vi "SPINUPGUN.vi"(10 "argv":string[](array[string]), 11 "args":u8) -> ()   [LabVIEW 2011]
uses:
  <vilib>/Rock Robotics/WPI/DriverStation/WPI_DriverStationStatusErrorCache.ctl
  signals/Signal.ctl
  Auto_Conf.vi
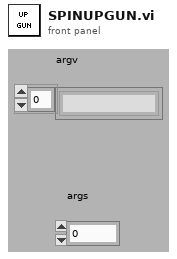
[diagram p1: front panel]
types:
  T1 = typedef "Signal.ctl" = enum16{"SIGFIRE", "SIGSTOPSCRIPT", "SIGSTARTGUN", "SIGSTOPGUN", "SIGDISABLED", "SIGENABLED", "SIGUDPTIMEOUT", "SIGNEWVISION_REMOTE", "SIGNEWVISION_LOCAL", "SIGSHOTFIRED", "SIGDOTRACK", "SIGDONTTRACK"}
  T2 = typedef "WPI_DriverStationStatusErrorCache.ctl" = enum16{"Get", "Set"}
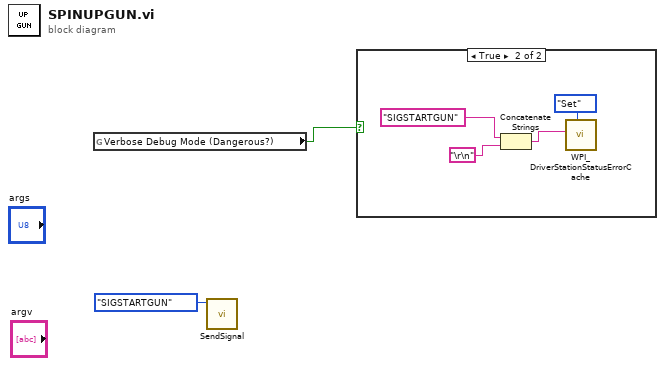
[diagram p0: block diagram]
diagram:
  n1 = global read "Auto_Conf.vi" "Verbose Debug Mode (Dangerous?)"() -> (w1:bool)
  n2 = call "SendSignal.vi"("Signal"=Signal."SIGSTARTGUN") -> ()  [unwired: 11 in]
  n3 = case shown="True" w1 {
    frame False {
    }
    frame True {
      n4 = Concatenate Strings("SIGSTARTGUN" ("string"), "\r\n") -> (w4:string)
      n5 = call <vilib>:"WPI_DriverStationStatusErrorCache.vi"("StatusErrorCacheOp"=WPI_DriverStationStatusErrorCache."Set", "Error String"=w4) -> ()  [unwired: 10 out]
    }
  }
